vi "create_icon.vi"(8 "error in (no error)":errorcluster, 9 "Icon File Path":path=path "C:/Program Files/National Instruments/LabVIEW 2009/applibs/lvapp.ico", 10 "Context Menu (optional)":string[][](array[string]), 11 "BalloonNotifier in":refnum<class "BalloonNotifier.lvclass">) -> (0 "error out":errorcluster, 3 "BalloonNotifier out":refnum<class "BalloonNotifier.lvclass">)   [LabVIEW 2017, in "BalloonNotifier.lvclass"]
uses:
  BalloonNotifier.lvclass
  BalloonNotifier.lvclass/BalloonNotifier.ctl
  System.Windows.Forms
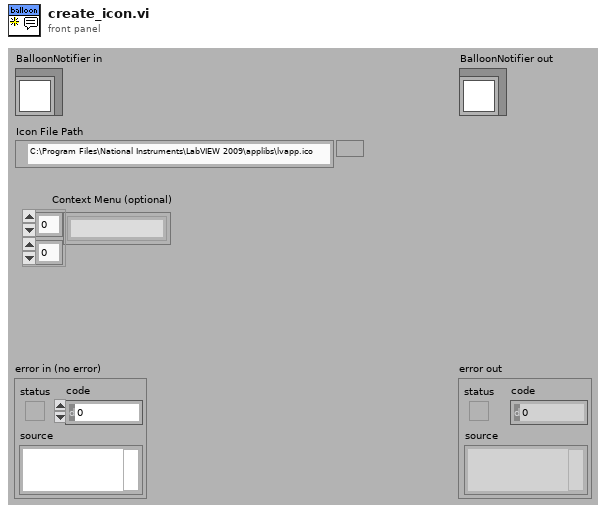
[diagram p1: front panel]
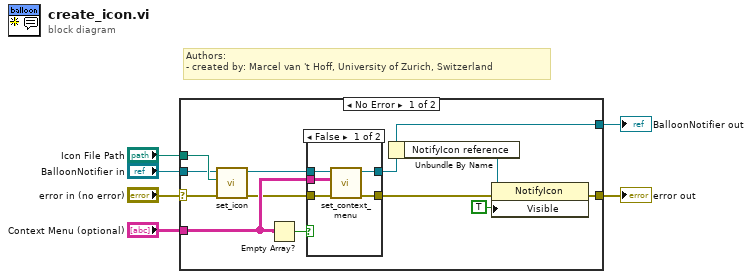
[diagram p0: block diagram]
diagram:
  # "Authors: \n- created by: Marcel van 't Hoff, University of Zurich, Switzerland"
  n1 = case shown="No Error" "error in (no error)" {
    selector: "error in (no error)" -> [w11 w27]
    tunnel: [w18 w27] -> w4
    tunnel: "Icon File Path" -> [w12 _]
    tunnel: "Context Menu (optional)" -> [w15 _]
    tunnel: "BalloonNotifier in" -> [w7 w26]
    tunnel: [w9 w26] -> w1
    frame No Error {
      n2 = call-dynamic "set_icon.vi"("error in (no error)"=w11, "Icon File Path"=w12, "BalloonNotifier in"=w7) -> ("error out"=w13:errorcluster, "BalloonNotifier out"=w10:refnum<class "BalloonNotifier.lvclass">)  [unwired: 7 in]
      n3 = Empty Array?(array=w15) -> (empty?=w14:bool)
      n4 = case shown="False" w14 {
        tunnel: w13 -> [w23 w25]
        tunnel: [w20 w25] -> w16
        tunnel: w15 -> [w22 _]
        tunnel: w10 -> [w21 w24]
        tunnel: [w19 w24] -> w9
        frame False {
          n5 = call-dynamic "set_context_menu.vi"("error in (no error)"=w23, "Context Menu"=w22, "BalloonNotifier in"=w21) -> ("error out"=w20:errorcluster, "BalloonNotifier out"=w19:refnum<class "BalloonNotifier.lvclass">)  [unwired: 7 in]
        }
        frame True {
        }
      }
      n6 = Unbundle By Name(w9) -> ("NotifyIcon reference"=w8:refnum<k24>)
      n7 = property class="NotifyIcon"(reference=w8, error in=w16, "Visible"=TRUE) -> (error out=w18:errorcluster)  [unwired: 1 out]
    }
    frame Error {
    }
  }
  "error out" <- w4
  "BalloonNotifier out" <- w1
